vi "testGetSubArray.vi"(8 "error in (no error)":errorcluster) -> (0 "error out":errorcluster)   [LabVIEW 2016]
doc: "Test to get the sub-array."
uses:
  MatOper/getSubArray1D.vi
  MatOper/getSubArray2D.vi
  MatOper/getSubArray3D.vi
  <vilib>/addons/_JKI Toolkits/Caraya/classes/Assert/Assert.lvclass
  <vilib>/addons/_JKI Toolkits/Caraya/classes/Test/Test.lvclass
  MatOper/MatOper.lvclass
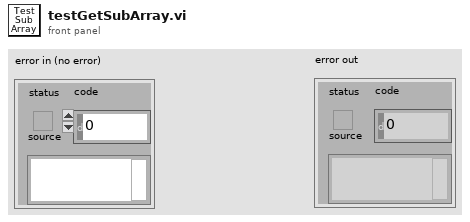
[diagram p1: front panel]
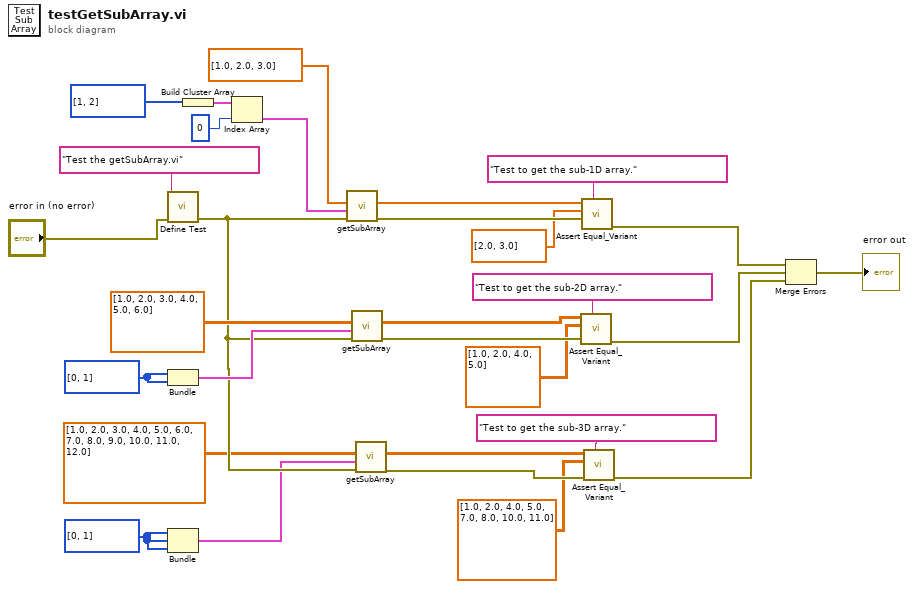
[diagram p0: block diagram]
diagram:
  w7 = i32[] [0, 1]
  w18 = i32[] [0, 1]
  n1 = call <vilib>:"Define Test.vi"("error in (no error)"="error in (no error)", "Label (VI Title)"="Test the getSubArray.vi") -> ("error out"=w9:errorcluster)  [unwired: 9 in]
  n2 = Bundle(w18, w18) -> (w17:cluster{i32[], i32[]})  [unwired: 1 in]
  n3 = Bundle(w7, w7, w7) -> (w6:cluster{i32[], i32[], i32[]})  [unwired: 1 in]
  n4 = Build Cluster Array(i32[] [1, 2]) -> (w24:cluster{i32[]}[])
  n5 = Index Array(array=w24, index=0) -> (element=w21:cluster{i32[]})
  n6 = call-poly "getSubArray.vi"("error in (no error)"=w9, "Index Array Cluster"=w21, "1D Array"=dbl[] [1.0, 2.0, 3.0]) -> ("error out"=w26:errorcluster, "Sub-Array"=w25:dbl[])  [unwired: 6 in, 1 out]
  n7 = call-poly "getSubArray.vi"("error in (no error)"=w9, "Index Array Cluster"=w17, "2D Array"=dbl[][] [[1.0, 2.0, 3.0], [4.0, 5.0, 6.0]]) -> ("error out"=w16:errorcluster, "Sub-Array"=w15:dbl[][])  [unwired: 6 in, 1 out]
  n8 = call-poly "getSubArray.vi"("error in (no error)"=w9, "Index Array Cluster"=w6, "3D Array"=dbl[][][] [[[1.0, 2.0, 3.0], [4.0, 5.0, 6.0]], [[7.0, 8.0, 9.0], [10.0, 11.0, 12.0]]]) -> ("error out"=w4:errorcluster, "Sub-Array"=w5:dbl[][][])  [unwired: 6 in, 1 out]
  n9 = call <vilib>:"Assert Equal_Variant.vi"("Label"="Test to get the sub-2D array.", "error in (no error)"=w16, "Y"=dbl[][] [[1.0, 2.0], [4.0, 5.0]], "X"=w15) -> ("error out"=w11:errorcluster)  [unwired: 7 in]
  n10 = call <vilib>:"Assert Equal_Variant.vi"("Label"="Test to get the sub-1D array.", "error in (no error)"=w26, "Y"=dbl[] [2.0, 3.0], "X"=w25) -> ("error out"=w12:errorcluster)  [unwired: 7 in]
  n11 = call <vilib>:"Assert Equal_Variant.vi"("Label"="Test to get the sub-3D array.", "error in (no error)"=w4, "Y"=dbl[][][] [[[1.0, 2.0], [4.0, 5.0]], [[7.0, 8.0], [10.0, 11.0]]], "X"=w5) -> ("error out"=w3:errorcluster)  [unwired: 7 in]
  n12 = Merge Errors(w12, w11, w3) -> (→"error out":errorcluster)
